vi "lab11.vi"() -> ()   [LabVIEW 2017]
uses:
  <vilib>/sound2/lvsound2.llb/Sound Data Format.ctl
  Control 1.ctl
  set_get.ctl
  <vilib>/sound2/lvsound2.llb/Sampling Mode.ctl
  <vilib>/measure/maspectr.llb/FFT Power Spectrum and PSD for N Chan.vi
  <vilib>/sound2/lvsound2.llb/Sound Input Read (DBL).vi
  <vilib>/measure/NI_MAPro.lvlib
panel:
  in  "stop":bool
  in  "Play":bool
  out "Power spectrum":cluster{"f0":dbl, "df":dbl, "magnitude":dbl[]}[](graph)
  in  "number of samples/ch 2":i32=100000
  in  "sound format":T1={"sample rate (S/s)"=22050.0, "number of channels"=2, "bits per sample"=16}
  out "Time Signal":waveform(dbl)[](graph)
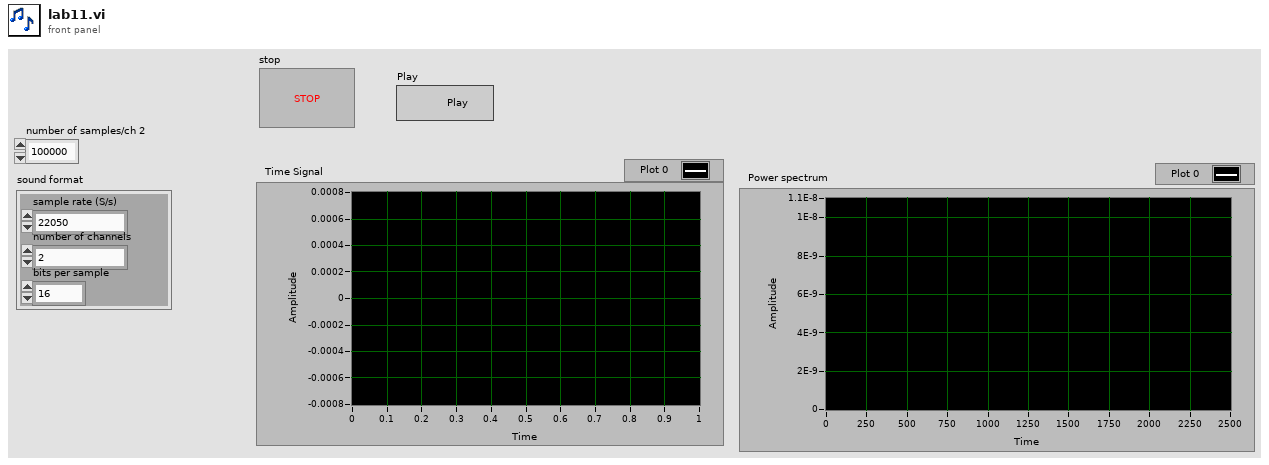
[diagram p1: front panel]
types:
  T1 = typedef "Sound Data Format.ctl" = cluster{"sample rate (S/s)":dbl, "number of channels":i32, "bits per sample":i32}
  T2 = typedef "Control 1.ctl" = enum16{"Idle", "Initialization", "Aquisition", "End"}
  T3 = typedef "set_get.ctl" = enum16{"set", "get"}
  T4 = cluster{"number of samples/ch 2":i32, "Play":bool, "sound format":T1}
  T5 = cluster{"number of samples/ch 2":i32, bool, "sound format":T1}
  T6 = typedef "Sampling Mode.ctl" = i32
  T7 = typedef "Sound Input Task ID.ctl" = u32
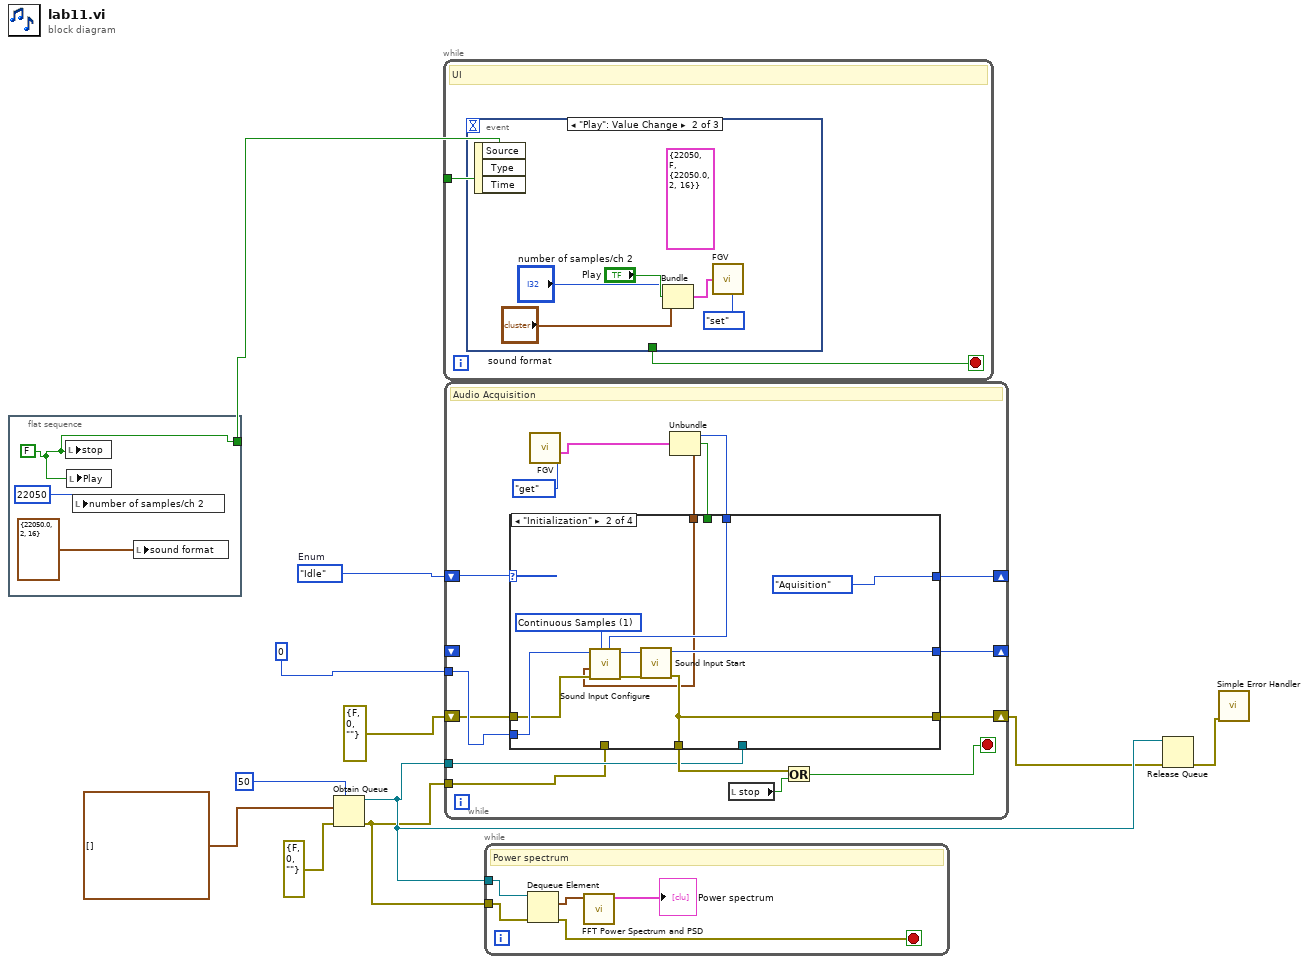
[diagram p0: block diagram]
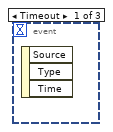
[diagram p2: hidden frame]
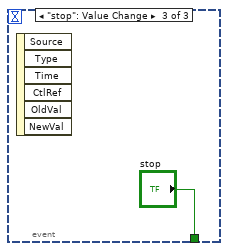
[diagram p3: hidden frame]
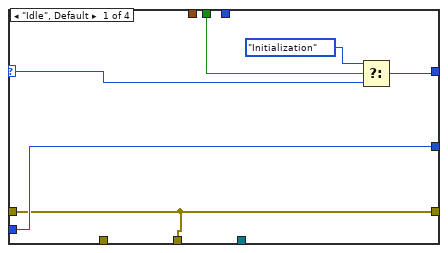
[diagram p4: hidden frame]
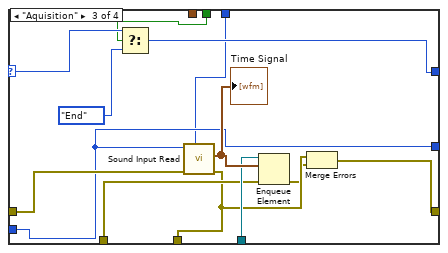
[diagram p5: hidden frame]
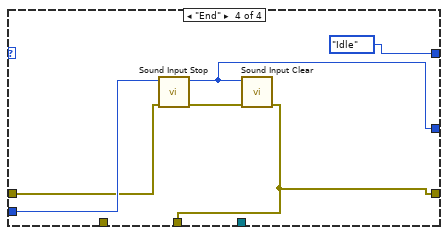
[diagram p6: hidden frame]
diagram:
  w10 = Control_1."Idle"  # Enum
  n1 = flat-sequence {
    tunnel: [w12] -> w3
    frame #0 {
      w12 = FALSE ("stop")
      n2 = local write "stop"(w12) -> ()
      n3 = local write "Play"(w12) -> ()
      n4 = local write "number of samples/ch 2"(22050 ("number of samples/ch 2")) -> ()
      n5 = local write "sound format"(T1 {"sample rate (S/s)"=22050.0, "number of channels"=2, "bits per sample"=16} ("sound format")) -> ()
    }
  }
  n6 = Obtain Queue(max queue size (-1, unlimited)=50, element data type=waveform(dbl)[] [] ("data"), error in (no error)=errorcluster {"status"=FALSE, "code"=0, "source"=""}) -> (queue out=w5:refnum<queue>, error out=w4:errorcluster)  [unwired: 2 in, 1 out]
  n7 = while {
    tunnel: w3 -> [_]
    stop <- w15 stop-if-true
    # "UI"
    n8 = event shown="[1] \"Play\": Value Change" {
      selector: _ -> [_ _ _]
      dyn-events: _ -> [_ _ _]
      timeout: _ -> [_ _ _]
      tunnel: [_ _ "stop"] -> w15
      event Timeout {
        n9 = event-data() -> ()  [unwired: 1 in, 3 out]
      }
      event "Play": Value Change {
        (unwired) T4 {"number of samples/ch 2"=22050, "Play"=FALSE, "sound format"={"sample rate (S/s)"=22050.0, "number of channels"=2, "bits per sample"=16}} ("cluster")
        n10 = event-data() -> ()  [unwired: 1 in, 3 out]
        n11 = Bundle("number of samples/ch 2"="number of samples/ch 2", "Play"="Play", "sound format"="sound format") -> (w17:T4)  [unwired: 1 in]
        n12 = call "FGV.vi"("Enum"=set_get."set", "Param In"=w17) -> ()  [unwired: 5 in, 1 out]
      }
      event "stop": Value Change {
        n13 = event-data() -> ()  [unwired: 1 in, 6 out]
      }
    }
  }
  n14 = while {
    shift-right: [w36] -> _
    shift-left: w10 -> [w33]
    shift-right: [w35] -> w2
    shift-left: errorcluster {"status"=FALSE, "code"=0, "source"=""} ("error in (no error)") -> [w29]
    shift-right: [w34] -> _
    shift-left: _ -> [_]
    tunnel: w5 -> [w32]
    tunnel: w4 -> [w31]
    tunnel: u32 0 ("device ID") -> [w30]
    stop <- w28 stop-if-true
    # "Audio Acquisition"
    n15 = call "FGV.vi"("Enum"=set_get."get") -> ("Param Out"=w25:T5)  [unwired: 6 in]
    n16 = Unbundle(w25) -> ("number of samples/ch 2"=w23:i32, w24:bool, "sound format"=w22:T1)
    n17 = case shown="\"Initialization\"" w33 {
      selector: w33 -> [w41 _ w64 _]
      tunnel: [w43 Control_1."Aquisition" ("Enum") w65 Control_1."Idle" ("Enum")] -> w36
      tunnel: [w39 w53 w58 w70] -> w37
      tunnel: [w39 w53 w56 w70] -> w35
      tunnel: [w40 w52 w59 w71] -> w34
      tunnel: w30 -> [w40 w48 w59 w68]
      tunnel: w32 -> [_ _ w62 _]
      tunnel: w31 -> [_ _ w61 _]
      tunnel: w29 -> [w39 w47 w60 w67]
      tunnel: w24 -> [w38 _ w55 _]
      tunnel: w23 -> [_ w45 w54 _]
      tunnel: w22 -> [_ w44 _ _]
      frame "Idle", Default {
        n18 = Select(t=Control_1."Initialization" ("Enum"), s=w38, f=w41) -> (s? t:f=w43:T2)
      }
      frame "Initialization" {
        w46 = T6 1 items=["Finite Samples", "Continuous Samples"] ("sample mode")
        n19 = call <vilib>:"Sound Input Configure.vi"("number of samples/ch"=w45, "sample mode"=w46, "error in (no error)"=w47, "sound format"=w44, "device ID"=w48) -> ("error out"=w49:errorcluster, "task ID"=w50:T7)  [unwired: 5 in]
        n20 = call <vilib>:"Sound Input Start.vi"("error in (no error)"=w49, "task ID"=w50) -> ("error out"=w53:errorcluster, "task ID out"=w52:T7)  [unwired: 8 in]
      }
      frame "Aquisition" {
        n21 = Select(t=w64, s=w55, f=Control_1."End" ("Enum")) -> (s? t:f=w65:T2)
        n22 = call-poly <vilib>:"Sound Input Read.vi"("number of samples/ch"=w54, "error in (no error)"=w60, "task ID"=w59) -> ("error out"=w58:errorcluster, "data"=w63:waveform(dbl)[])  [unwired: 6 in, 1 out]
        "Time Signal" <- w63
        n23 = Enqueue Element(queue=w62, element=w63, error in (no error)=w61) -> (error out=w57:errorcluster)  [unwired: 1 in, 2 out]
        n24 = Merge Errors(w58, w57) -> (w56:errorcluster)
      }
      frame "End" {
        n25 = call <vilib>:"Sound Input Stop.vi"("error in (no error)"=w67, "task ID"=w68) -> ("error out"=w72:errorcluster, "task ID out"=w71:T7)  [unwired: 8 in]
        n26 = call <vilib>:"Sound Input Clear.vi"("error in (no error)"=w72, "task ID"=w71) -> ("error out"=w70:errorcluster)  [unwired: 9 in]
      }
    }
    n27 = local read "stop"() -> (w27:bool)
    n28 = Or(x=w37, y=w27) -> (x .or. y?=w28:bool)
  }
  n29 = while {
    tunnel: w5 -> [w76]
    tunnel: w4 -> [w75]
    stop <- w73 stop-if-true
    # "Power spectrum"
    n30 = Dequeue Element(queue=w76, error in (no error)=w75) -> (element=w74:waveform(dbl)[], error out=w73:errorcluster)  [unwired: 1 in, 2 out]
    n31 = call-poly <vilib>:"FFT Power Spectrum and PSD.vi"("time signals"=w74) -> ("Power Spectrum / PSD"=→"Power spectrum":cluster{"f0":dbl, "df":dbl, "magnitude":dbl[]}[])  [unwired: 7 in, 3 out]
  }
  n32 = Release Queue(queue=w5, error in (no error)=w2) -> (error out=w1:errorcluster)  [unwired: 1 in, 2 out]
  n33 = call <vilib>:"Simple Error Handler.vi"("error in (no error)"=w1) -> ()  [unwired: 4 in, 5 out]
